vi "Read Array.vi"(11 "Double Array Event in":refnum<class "Double Array Event.lvclass">) -> (2 "Array":dbl[](array[numeric]), 3 "Double Array Event out":refnum<class "Double Array Event.lvclass">)   [LabVIEW 2016, in "Double Array Event.lvclass"]
uses:
  Double Array Event.lvclass
  Double Array Event.lvclass/Double Array Event.ctl
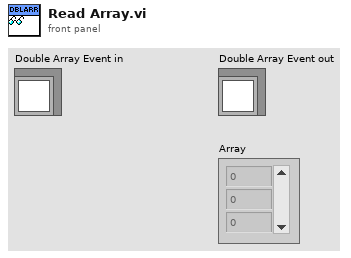
[diagram p1: front panel]
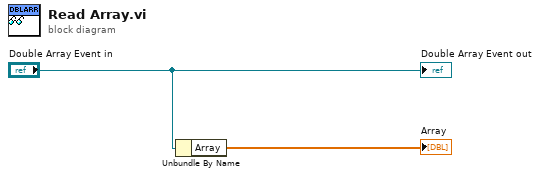
[diagram p0: block diagram]
diagram:
  n1 = Unbundle By Name("Double Array Event in") -> ("Array"=→"Array":dbl[])
  "Double Array Event out" <- "Double Array Event in"
